vi "Looper.vi"() -> ()   [LabVIEW 2018]
uses:
  <vilib>/imath/engines/lvmath2/RunTimeEngine/NodeEndStatement/NIMS_NodeEndStatement_Output.vi
  <instcachedir>/0/NIMS_NodeEndStatement_Output_53EC0D466D134D7ABD903AC30B43404B.lvgen/NIMS_NodeEndStatement_Output_53EC0D466D134D7ABD903AC30B43404B_005.vi
  <vilib>/imath/engines/lvmath2/RunTimeEngine/ErrorHandling/NIMS_Finalize Error.vi
  <vilib>/Utility/file.llb/Write Delimited Spreadsheet (DBL).vi
panel:
  in  "File Name":string
  in  "String 2":string="bpm.txt"
  in  "String 1":string="Impedance_Jeff_"
  out "Impedance (Phase)":cluster{dbl[], dbl[]}(graph)
  out "Impedance (Mag)":cluster{dbl[], dbl[]}(graph)
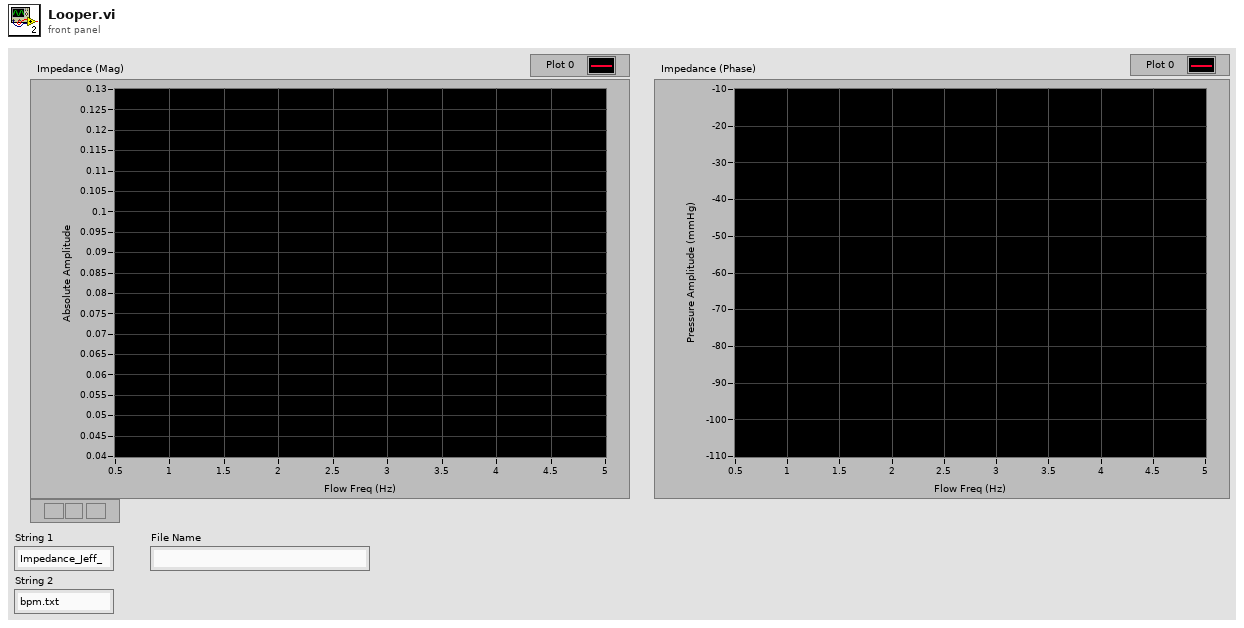
[diagram p1: front panel]
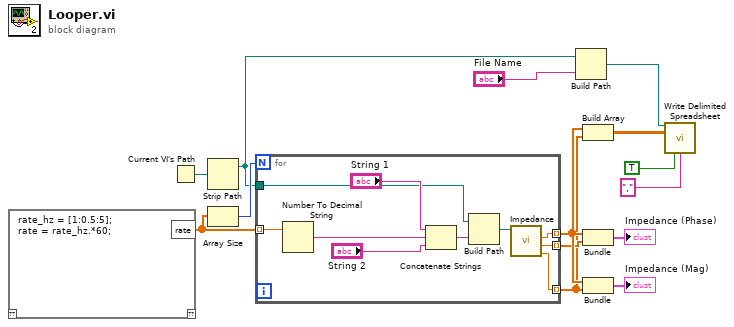
[diagram p0: block diagram]
diagram:
  n1 = mathscript code="rate_hz = [1:0.5:5];\nrate = rate_hz.*60;"() -> ("rate"=w13:dbl[])  [unwired: 1 in, 1 out]
  n2 = Current VI's Path() -> (path=w12:path)
  n3 = Strip Path(path=w12) -> (stripped path=w5:path)  [unwired: 1 out]
  n4 = Array Size(array=w13) -> (size(s)=w14:i32)
  n5 = for {
    N: w14 -> [_]
    tunnel: w13 -> [w24] mode=indexing
    tunnel: [w20] -> w11 mode=indexing
    tunnel: w5 -> [w17]
    tunnel: [w16] -> w10 mode=indexing
    tunnel: [w15] -> w8 mode=indexing
    n6 = Number To Decimal String(number=w24) -> (decimal integer string=w22:string)  [unwired: 1 in]
    n7 = Concatenate Strings("String 1", w22, "String 2") -> (w19:string)
    n8 = Build Path(base path=w17, name or relative path=w19) -> (appended path=w18:path)
    n9 = call "Impedance.vi"("file path (dialog if empty)"=w18) -> ("Abs Amplitude"=w15:dbl, "Phase (deg)"=w16:dbl, "Flow Freq (Hz)"=w20:dbl)  [unwired: 7 in, 1 out]
  }
  n10 = Build Path(base path=w5, name or relative path="File Name") -> (appended path=w1:path)
  n11 = Build Array(w11, w8) -> (w4:dbl[][])
  n12 = Bundle(w11, w10) -> (→"Impedance (Phase)":cluster{dbl[], dbl[]})  [unwired: 1 in]
  n13 = Bundle(w11, w8) -> (→"Impedance (Mag)":cluster{dbl[], dbl[]})  [unwired: 1 in]
  n14 = call-poly <vilib>:"Write Delimited Spreadsheet.vi"("file path (dialog if empty)"=w1, "2D data"=w4, "transpose? (no:F)"=TRUE, "delimiter (\\t)"="," ("delimiter (\\t)")) -> ()  [unwired: 10 in, 2 out]
